vi "Turn Power Off Command.vi"(8 "error in (no error)":errorcluster, 11 "command_TurnPowerOff":T1) -> (0 "error out":errorcluster)   [LabVIEW 2016, in "M1M3SupportEUI_Views.lvlib"]
uses:
  M1M3SupportEUI_Views.lvlib
  SALLV_m1m3/DataTypes/command_TurnPowerOff.ctl
  SALLV_m1m3/SALLV_m1m3.lvlib
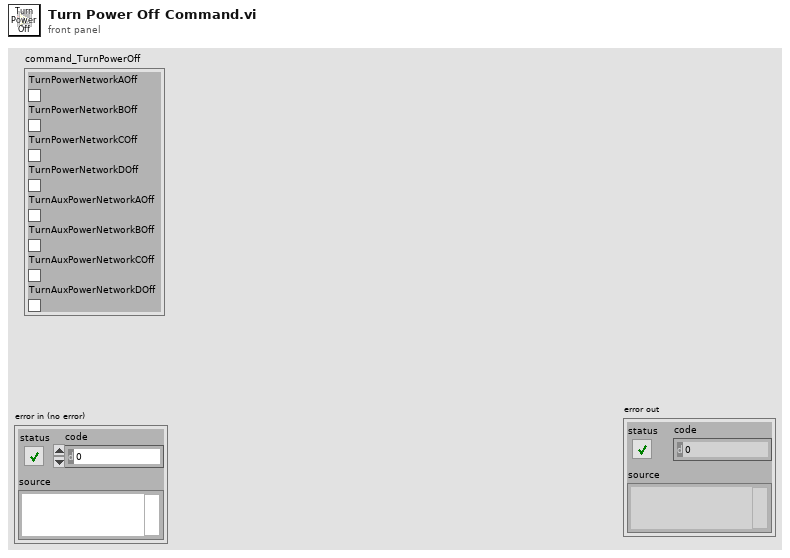
[diagram p1: front panel]
types:
  T1 = typedef "SALLV_m1m3.lvlib/command_TurnPowerOff.ctl" = cluster{"TurnPowerNetworkAOff":bool, "TurnPowerNetworkBOff":bool, "TurnPowerNetworkCOff":bool, "TurnPowerNetworkDOff":bool, "TurnAuxPowerNetworkAOff":bool, "TurnAuxPowerNetworkBOff":bool, "TurnAuxPowerNetworkCOff":bool, "TurnAuxPowerNetworkDOff":bool}
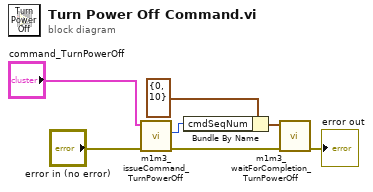
[diagram p0: block diagram]
diagram:
  n1 = call "m1m3_issueCommand_TurnPowerOff.vi"("error in (no error)"="error in (no error)", "command_TurnPowerOff_Ctl"="command_TurnPowerOff") -> ("error out"=w5:errorcluster, "function return"=w2:i32)  [unwired: 7 in, 1 out]
  n2 = Bundle By Name(cluster=cluster{"cmdSeqNum":i32, "timeout":u32} {"cmdSeqNum"=0, "timeout"=10} ("waitComplete_Ctl"), "cmdSeqNum"=w2) -> (w1:cluster{"cmdSeqNum":i32, "timeout":u32})
  n3 = call "m1m3_waitForCompletion_TurnPowerOff.vi"("error in (no error)"=w5, "waitComplete_Ctl"=w1) -> ("error out"=→"error out":errorcluster)  [unwired: 7 in, 2 out]
